vi "Viewer Control - Add Actor.vi"(8 "error in":errorcluster, 10 "Stop Viewer Actor":refnum<class "Message Enqueuer.lvclass">, 11 "App Data in":T1) -> (0 "error out":errorcluster, 3 "App Data out":T1)   [LabVIEW 2019]
uses:
  <vilib>/ActorFramework/Message Enqueuer/Message Enqueuer.lvclass
  Typedefs/#cluster_ApplicationData.ctl
  Typedefs/Acquisition Thread/#cluster_AcqQueueData.ctl
  Typedefs/Acquisition Thread/#enum_AcquisitionTask.ctl
  Typedefs/Saving Thread/#cluster_SavingQueueData.ctl
  Typedefs/Saving Thread/#enum_SavingTask.ctl
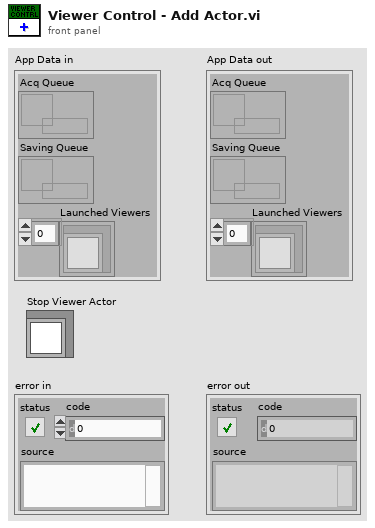
[diagram p1: front panel]
types:
  T1 = typedef "#cluster_ApplicationData.ctl" = cluster{"Acq Queue":refnum<queue>, "Saving Queue":refnum<queue>, "Launched Viewers":refnum<class "Message Enqueuer.lvclass">[]}
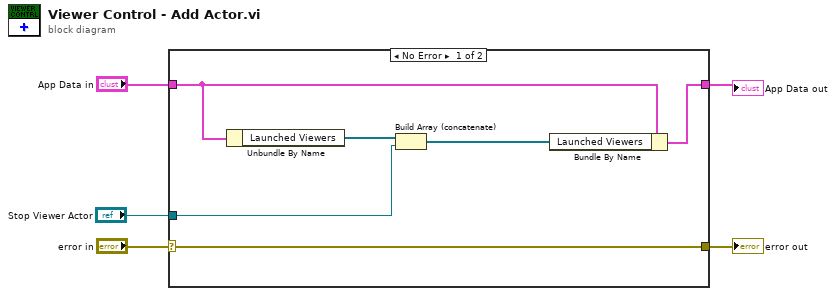
[diagram p0: block diagram]
diagram:
  n1 = case shown="No Error" "error in" {
    selector: "error in" -> [w9 w13]
    tunnel: [w11 w12] -> w5
    tunnel: "App Data in" -> [w10 w12]
    tunnel: [w9 w13] -> w2
    tunnel: "Stop Viewer Actor" -> [w7 _]
    frame No Error {
      n2 = Unbundle By Name(w10) -> ("Launched Viewers"=w8:refnum<class "Message Enqueuer.lvclass">[])
      n3 = Build Array (concatenate)(w8, w7) -> (w6:refnum<class "Message Enqueuer.lvclass">[])
      n4 = Bundle By Name(cluster=w10, "Launched Viewers"=w6) -> (w11:T1)
    }
    frame Error {
    }
  }
  "error out" <- w2
  "App Data out" <- w5
